vi "upgrade_load.vi"(5 "fator de kVAr":dbl, 7 "Quantity":string, 9 "Loads":string="  N0001A                  43264.275.42                                         0\n  N0002B                  86528.550.85                                         0\n  N0004C                  43264.275.42                                         0\n  N0005C                  86528.550.85                                         0\n  N0006C                  43264.275.42                                         0\n  N0007A                  86528.550.85                                         0\n  N0009A                  43264.275.42                                         0\n  N0010A                  86528.550.85                                         0\n  N0011A                  43264.275.42                                         0\n  N0012B                  86528.550.85                                         0\n  N0016C                  43264.275.42                                         0\n  N0017C                  86528.550.85                                         0\n  N0019A                  43264.275.42                                         0\n  N0020A                  43264.275.42                                         0\n  N0022B                  43264.275.42                                         0\n  N0024C                  43264.275.42                                         0\n  N0028A                  43264.275.42                                         0\n  N0029A                  43264.275.42                                         0\n  N0030C                  43264.275.42                                         0\n  N0031C                  86528.550.85                                         0\n  N0032C                  86528.550.85                                         0\n  N0033A                  43264.275.42                                         0\n  N0034C                  43264.275.42                                         0\n  N0035A                  43264.275.42                                         0\n  N0037A                  43264.275.42                                         0\n  N0038B                  86528.550.85                                         0\n  N0039B                  86528.550.85                                         0\n  N0041C                  86528.550.85                                         0\n  N0042A                  86528.550.85                                         0\n  N0043B                  43264.275.42                                         0\n  N0045A                  86528.550.85                                         0\n  N0046A                  86528.550.85                                         0\n  N0047A                  49444.220.34                                         0\n  N0047B                  49444.220.34                                         0\n  N0047C                  49444.220.34                                         0\n  N0048A                  24722.110.17                                         0\n  N0048B                  24722.110.17                                         0\n  N0048C                  24722.110.17                                         0\n  N0049A                  49444.220.34                                         0\n  N0049B                  24722.110.17                                         0\n  N0049C                  49444.275.42                                         0\n  N0050C                  43264.275.42                                         0\n  N0051A                  86528.550.85                                         0\n  N0052A                  43264.275.42                                         0\n  N0053A                  43264.275.42                                         0\n  N0055A                  86528.550.85                                         0\n  N0056B                  86528.550.85                                         0\n  N0058B                  86528.550.85                                         0\n  N0059B                  86528.550.85                                         0\n  N0060A                  86528.550.85                                         0\n  N0062C                  43264.275.42                                         0\n  N0063A                  43264.275.42                                         0\n  N0064B                  23074.157.38                                         0\n  N0065A                  49444.220.34                                         0\n  N0065B                  49444.220.34                                         0\n  N0065C                  24722.110.17                                         0\n  N0066C                  23074.157.38                                         0\n  N0068A                  86528.550.85                                         0\n  N0069A                  43264.275.42                                         0\n  N0070A                  86528.550.85                                         0\n  N0071A                  43264.275.42                                         0\n  N0073C                  43264.275.42                                         0\n  N0074C                  43264.275.42                                         0\n  N0075C                  43264.275.42                                         0\n  N0076A                  16481.68.856                                         0\n  N0076B                  24722.110.17                                         0\n  N0076C                  24722.110.17                                         0\n  N0077B                  43264.275.42                                         0\n  N0079A                  43264.275.42                                         0\n  N0080B                  43264.275.42                                         0\n  N0082A                  43264.275.42                                         0\n  N0083C                  86528.550.85                                         0\n  N0084C                  86528.550.85                                         0\n  N0085C                  43264.275.42                                         0\n  N0086B                  86528.550.85                                         0\n  N0087B                  43264.275.42                                         0\n  N0088A                  43264.275.42                                         0\n  N0090B                  43264.275.42                                         0\n  N0092C                  43264.275.42                                         0\n  N0094A                  43264.275.42                                         0\n  N0095B                  86528.550.85                                         0\n  N0096B                  86528.550.85                                         0\n  N0098A                  43264.275.42                                         0\n  N0099B                  43264.275.42                                         0\n  N0100C                  43264.275.42                                         0\n  N0102C                  86528.550.85                                         0\n  N0103C                  43264.275.42                                         0\n  N0104C                  43264.275.42                                         0\n  N0106B                  43264.275.42                                         0\n  N0107B                  43264.275.42                                         0\n  N0109A                  43264.275.42                                         0\n  N0111A                  86528.550.85                                         0\n  N0112A                  86528.550.85                                         0\n  N0113A                  43264.275.42                                         0\n  N0114A                  86528.550.85                                         0", 10 "Event type":string="LL", 11 "Node":string="1") -> (1 "Actual loads":string)   [LabVIEW 2020]
panel:
  out "concatenated string":string
  in  "voltage":dbl=4160.0
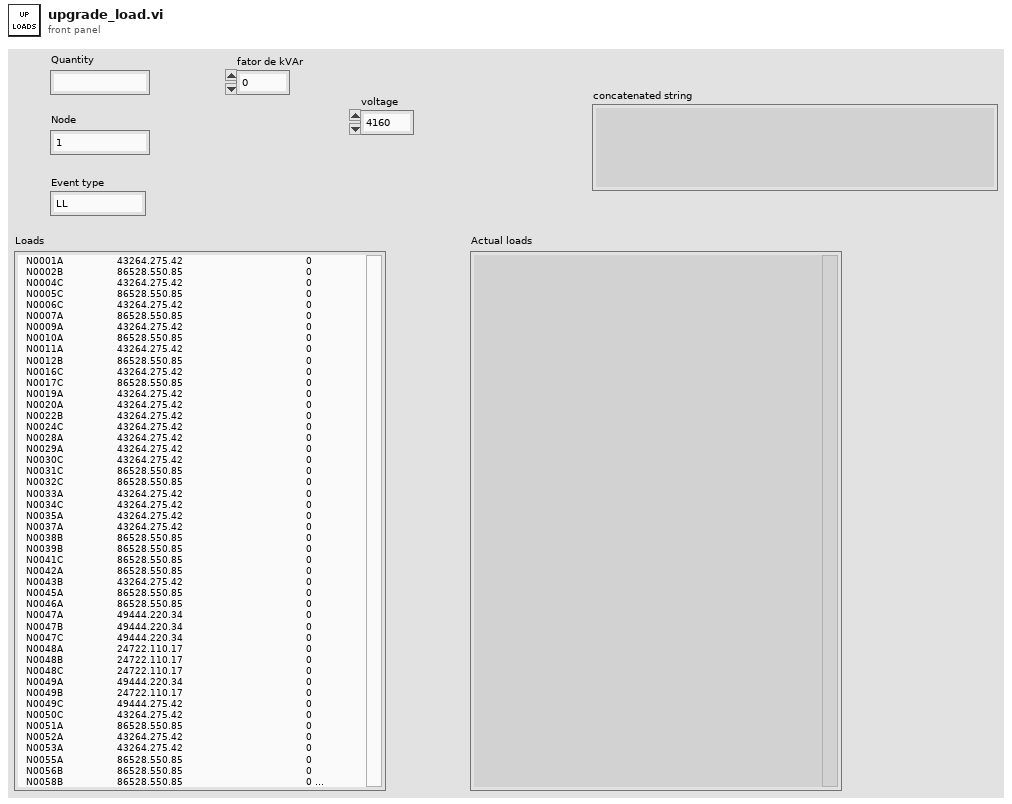
[diagram p1: front panel]
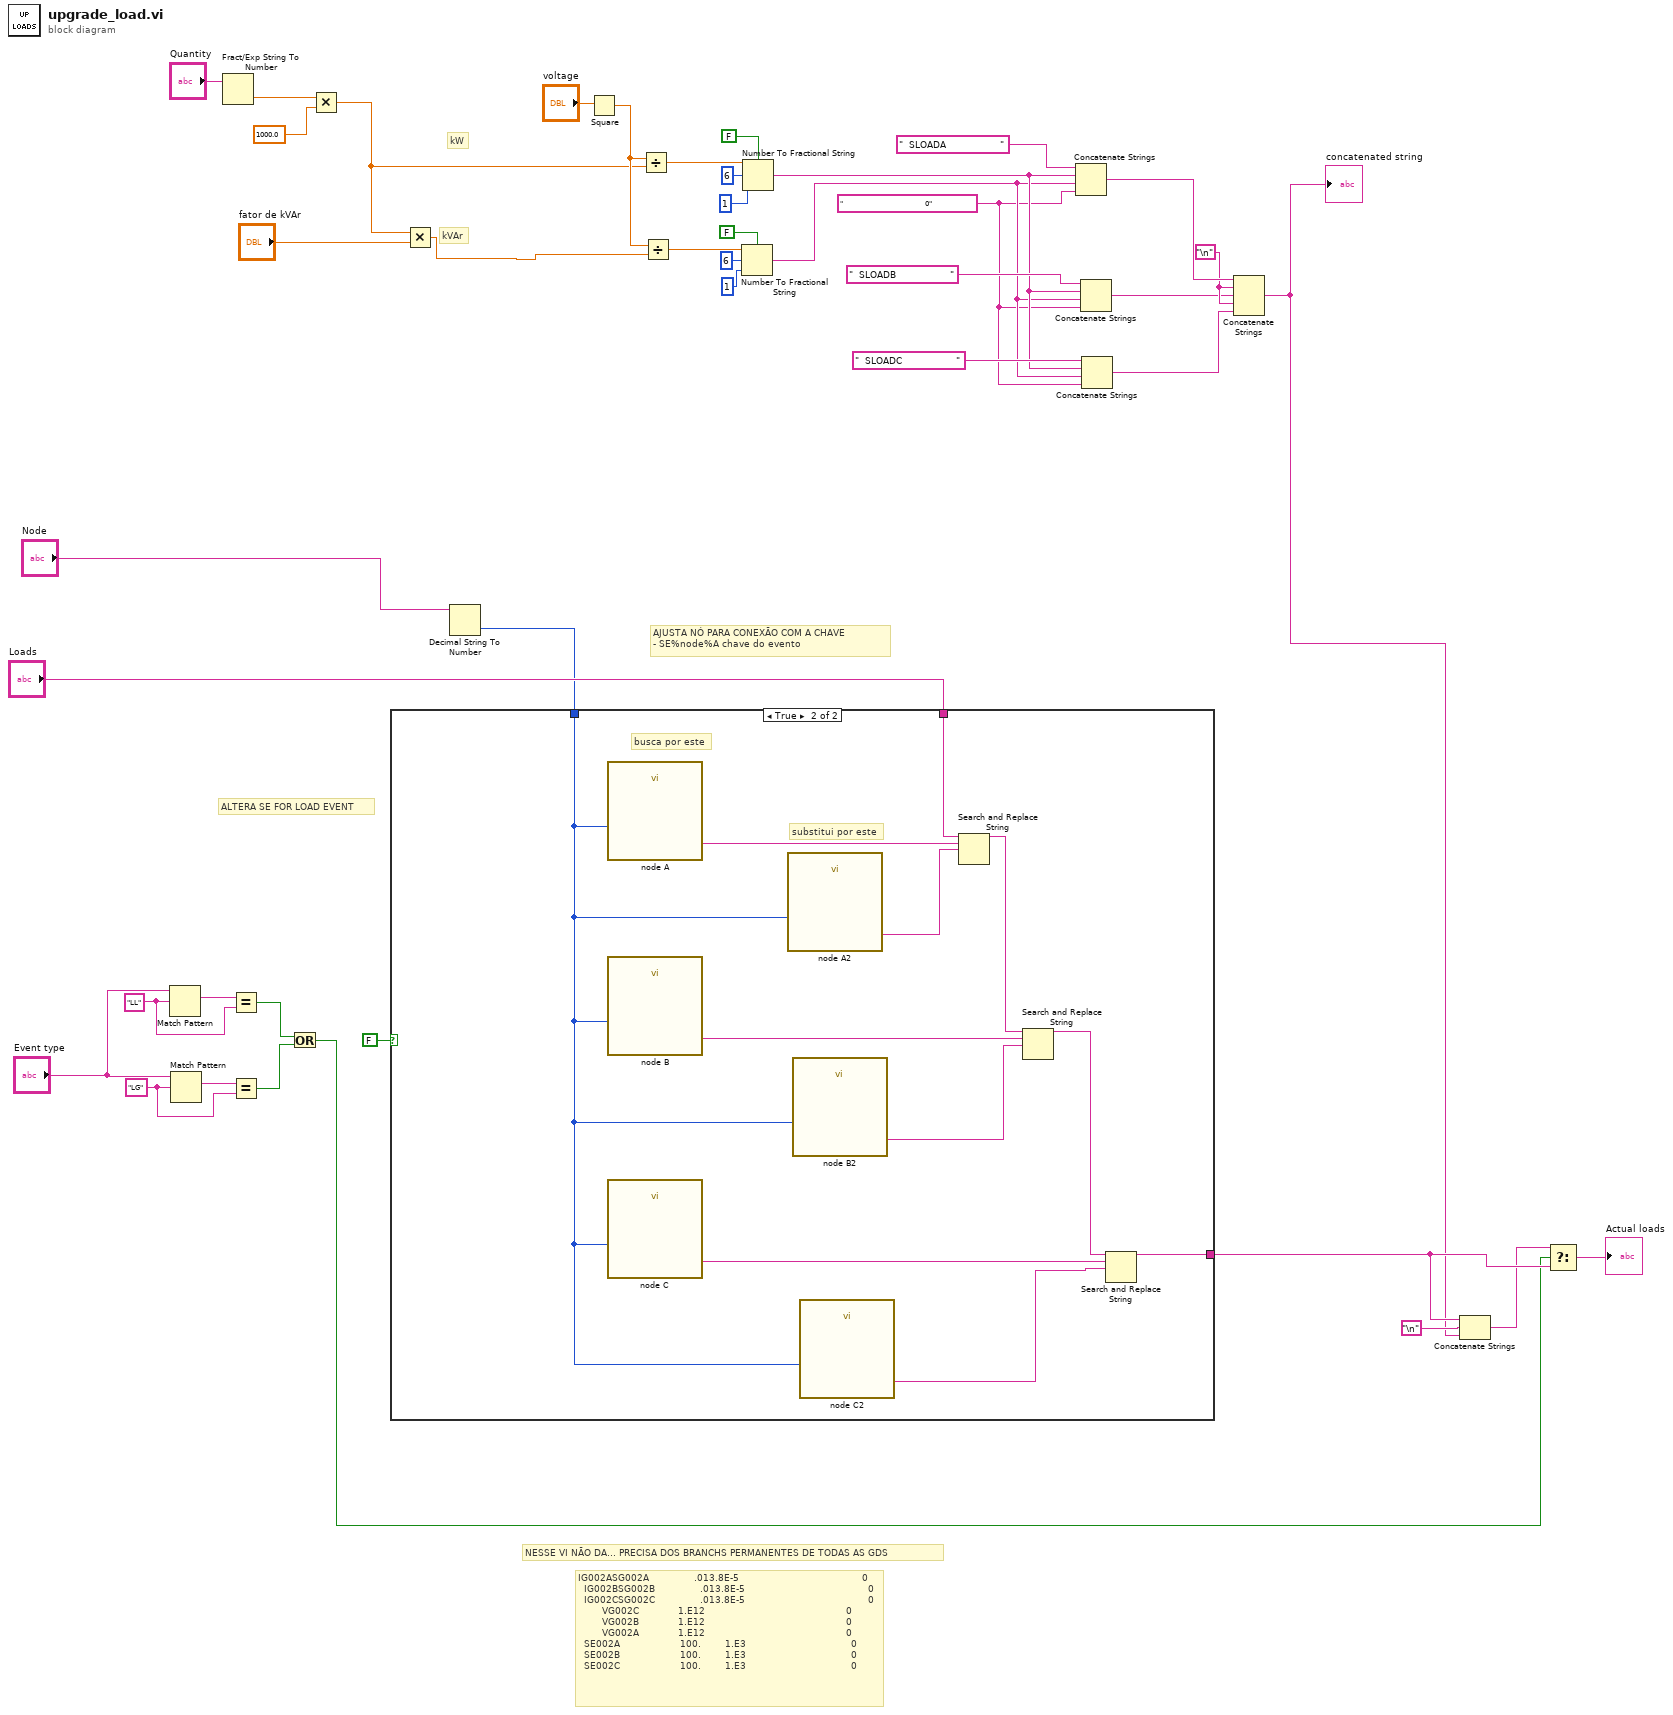
[diagram p0: block diagram]
diagram:
  w12 = "\n"
  w14 = "                                         0"
  w39 = "LL" ("regular expression")
  w37 = "LG" ("regular expression")
  # "kVAr"
  # "kW"
  # "NESSE VI NÃO DA... PRECISA DOS BRANCHS PERMANENTES DE TODAS AS GDS"
  # "IG002ASG002A               .013.8E-5                                         0\n  IG002BSG002B               .013.8E-5                                         0\n  IG002CSG002C               .013.8E-5                                         0\n        VG002C             1.E12                                               0\n        VG002B             1.E12                                               0\n        VG002A             1.E12                                               0\n  SE002A                    100.        1.E3                                   0\n  SE002B                    100.        1.E3                                   0\n  SE002C                    100.        1.E3                                   0"
  # "ALTERA SE FOR LOAD EVENT"
  # "AJUSTA NÓ PARA CONEXÃO COM A CHAVE\n- SE%node%A chave do evento"
  n1 = Match Pattern(string="Event type", regular expression=w39) -> (match substring=w38:string)  [unwired: 1 in, 3 out]
  n2 = Match Pattern(string="Event type", regular expression=w37) -> (match substring=w40:string)  [unwired: 1 in, 3 out]
  n3 = Fract/Exp String To Number(string="Quantity") -> (number=w4:dbl)  [unwired: 3 in, 1 out]
  n4 = Equal?(x=w38, y=w39) -> (x = y?=w35:bool)
  n5 = Equal?(x=w40, y=w37) -> (x = y?=w36:bool)
  n6 = Or(x=w35, y=w36) -> (x .or. y?=w30:bool)
  n7 = Multiply(x=w4, y=1000.0) -> (x*y=w1:dbl)
  n8 = Multiply(x=w1, y="fator de kVAr") -> (x*y=w2:dbl)
  n9 = Decimal String To Number(string="Node") -> (number=w41:i32)  [unwired: 2 in, 1 out]
  n10 = case shown="True" FALSE {
    tunnel: "Loads" -> [w44 w48]
    tunnel: [w44 w53] -> w33
    tunnel: w41 -> [_ w50]
    frame False {
    }
    frame True {
      # "substitui por este"
      # "busca por este"
      n11 = call "node A"("node"=w50) -> ("Result"=w47:string)  [unwired: 13 in, 1 out]
      n12 = call "node B"("node"=w50) -> ("Result"=w45:string)  [unwired: 13 in, 1 out]
      n13 = call "node C"("node"=w50) -> ("Result"=w55:string)  [unwired: 13 in, 1 out]
      n14 = call "node A2"("node"=w50) -> ("Result"=w52:string)  [unwired: 13 in, 1 out]
      n15 = call "node B2"("node"=w50) -> ("Result"=w51:string)  [unwired: 13 in, 1 out]
      n16 = call "node C2"("node"=w50) -> ("Result"=w49:string)  [unwired: 13 in, 1 out]
      n17 = Search and Replace String(input string=w48, search string=w47, replace string=w52) -> (result string=w46:string)  [unwired: 5 in, 3 out]
      n18 = Search and Replace String(input string=w46, search string=w45, replace string=w51) -> (result string=w54:string)  [unwired: 5 in, 3 out]
      n19 = Search and Replace String(input string=w54, search string=w55, replace string=w49) -> (result string=w53:string)  [unwired: 5 in, 3 out]
    }
  }
  n20 = Square(x="voltage") -> (x^2=w28:dbl)
  n21 = Divide(x=w28, y=w1) -> (x/y=w27:dbl)
  n22 = Divide(x=w28, y=w2) -> (x/y=w25:dbl)
  n23 = Number To Fractional String(use system decimal point (T)=FALSE, number=w25, width (-)=i16 6, precision (6)=i16 1) -> (F-format string=w15:string)
  n24 = Number To Fractional String(use system decimal point (T)=FALSE, number=w27, width (-)=i16 6, precision (6)=i16 1) -> (F-format string=w16:string)
  n25 = Concatenate Strings("  SLOADA                  ", w16, w15, w14) -> (w13:string)
  n26 = Concatenate Strings("  SLOADB                  ", w16, w15, w14) -> (w11:string)
  n27 = Concatenate Strings("  SLOADC                  ", w16, w15, w14) -> (w10:string)
  n28 = Concatenate Strings(w13, w12, w11, w12, w10) -> (w9:string)
  "concatenated string" <- w9
  n29 = Concatenate Strings(w33, "\n", w9) -> (w31:string)
  n30 = Select(t=w31, s=w30, f=w33) -> (s? t:f=→"Actual loads":string)
